vi "Get Wash State From Variant.vi"(8 "error in":errorcluster, 11 "Message Queue Data":T3) -> (0 "error out":errorcluster, 3 "WashState out":T1)   [LabVIEW 2018]
uses:
  MessageQueueData.ctl
  Command.ctl
  WashState.ctl
  Position.ctl
panel:
  in  "WashState in":T1
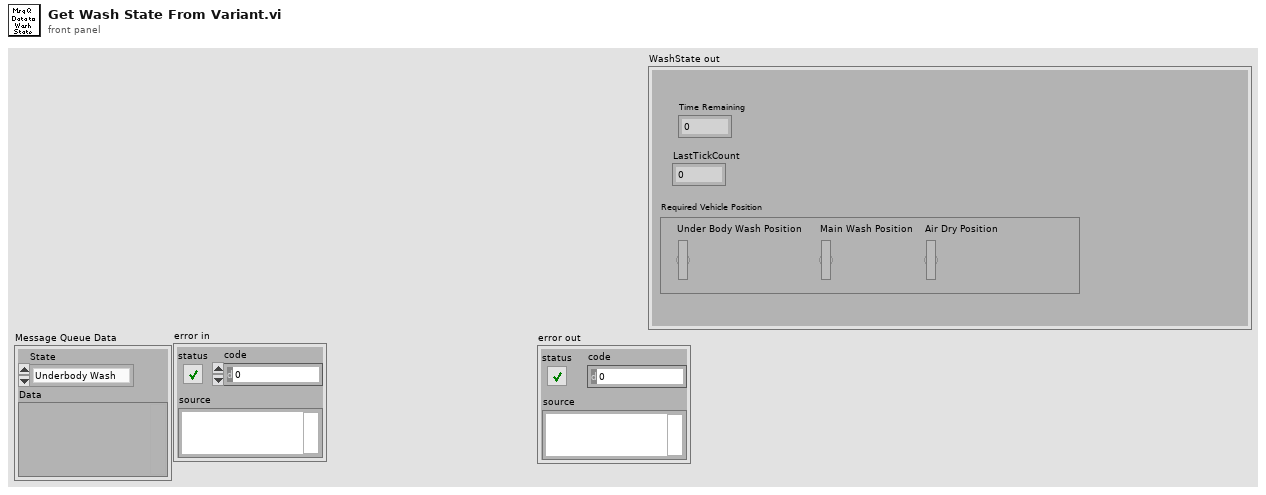
[diagram p1: front panel]
types:
  T1 = typedef "WashState.ctl" = cluster{"Time Remaining":i32, "LastTickCount":i32, "Required Vehicle Position":T2}
  T2 = typedef "Position.ctl" = enum32{"Under Body Wash Position", "Main Wash Position", "Air Dry Position"}
  T3 = typedef "MessageQueueData.ctl" = cluster{"State":T4, "Data":variant}
  T4 = typedef "Command.ctl" = enum16{"Underbody Wash", "Soap Application", "Main High-Pressure Wash", "Clear Water Rinse", "Air Dry Cycle", "Stop"}
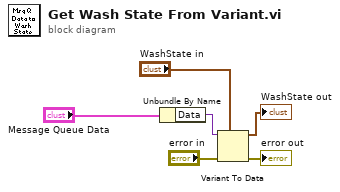
[diagram p0: block diagram]
diagram:
  n1 = Unbundle By Name("Message Queue Data") -> ("Data"=w4:variant)
  n2 = Variant To Data(error in="error in", type="WashState in", Variant=w4) -> (data=→"WashState out":T1, error out=→"error out":errorcluster)
